vi "Config Controller.vi"(6 "Corrente Limite (mA)":i32=500, 7 "Limite de Temperatura":dbl=27.0, 8 "error in (no error)":errorcluster, 9 "Corrente Inicial (mA)":dbl, 10 "Temperatura":dbl=25.0, 11 "VISA Refnum in":refnum<visa-resource-name>="GPIB0::1::INSTR") -> (0 "error out":errorcluster, 3 "VISA Refnum out":refnum<visa-resource-name>)   [LabVIEW 2021]
uses:
  9b799e5e-0c55-4328-8756-1c7587b2fd8d.vi
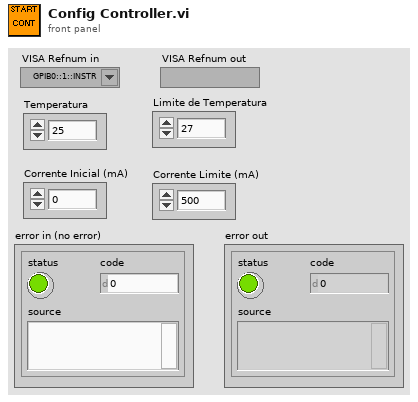
[diagram p1: front panel]
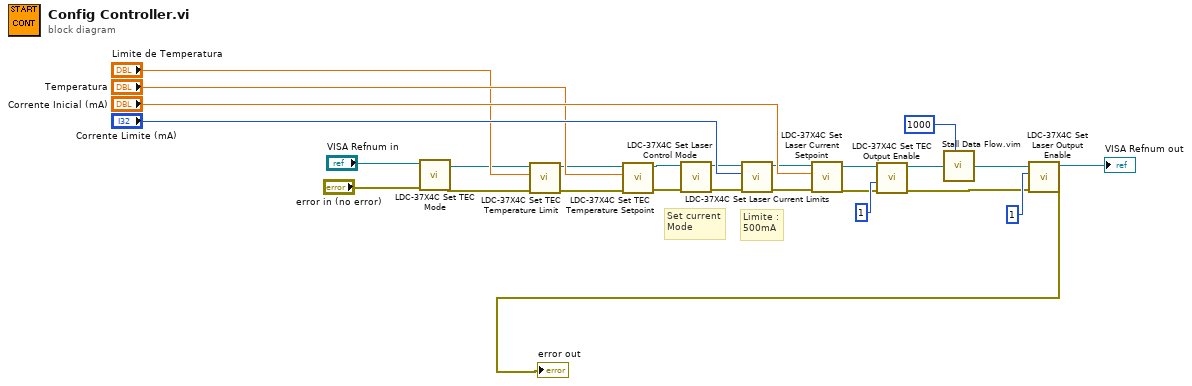
[diagram p0: block diagram]
diagram:
  # "Set current\nMode"
  # "Limite :\n500mA"
  n1 = call "LDC-37X4C Set TEC Mode.vi"("error in (no error)"="error in (no error)", "VISA resource name"="VISA Refnum in") -> ("error out"=w4:errorcluster, "VISA resource name out"=w3:refnum<visa-resource-name>)  [unwired: 8 in]
  n2 = call "LDC-37X4C Set TEC Temperature Limit.vi"("error in (no error)"=w4, "Limit"="Limite de Temperatura", "VISA resource name"=w3) -> ("error out"=w6:errorcluster, "VISA resource name out"=w5:refnum<visa-resource-name>)  [unwired: 7 in]
  n3 = call "LDC-37X4C Set TEC Temperature Setpoint.vi"("error in (no error)"=w6, "Temperature"="Temperatura", "VISA resource name"=w5) -> ("error out"=w8:errorcluster, "VISA resource name out"=w7:refnum<visa-resource-name>)  [unwired: 7 in]
  n4 = call "LDC-37X4C Set Laser Control Mode.vi"("error in (no error)"=w8, "VISA resource name"=w7) -> ("error out"=w11:errorcluster, "VISA resource name out"=w12:refnum<visa-resource-name>)  [unwired: 8 in]
  n5 = call "LDC-37X4C Set Laser Current Limits.vi"("error in (no error)"=w11, "Limit"="Corrente Limite (mA)", "VISA resource name"=w12) -> ("error out"=w10:errorcluster, "VISA resource name out"=w9:refnum<visa-resource-name>)  [unwired: 7 in]
  n6 = call "LDC-37X4C Set Laser Current Setpoint.vi"("error in (no error)"=w10, "Current"="Corrente Inicial (mA)", "VISA resource name"=w9) -> ("error out"=w14:errorcluster, "VISA resource name out"=w13:refnum<visa-resource-name>)  [unwired: 7 in]
  n7 = call "LDC-37X4C Set TEC Output Enable.vi"("error in (no error)"=w14, "input 1"=1, "VISA resource name"=w13) -> ("error out"=w15:errorcluster, "VISA resource name out"=w18:refnum<visa-resource-name>)  [unwired: 7 in]
  n8 = call "Stall Data Flow.vim"("value in"=w18, "milliseconds to wait"=u32 1000) -> ("value out"=w19:refnum<visa-resource-name>)  [unwired: 1 out]
  n9 = call "LDC-37X4C Set Laser Output Enable.vi"("error in (no error)"=w15, "input 2"=1, "VISA resource name"=w19) -> ("error out"=→"error out":errorcluster, "VISA resource name out"=→"VISA Refnum out":refnum<visa-resource-name>)  [unwired: 7 in]
